vi "Import Export - Import from XML File.vi"(8 "error in":errorcluster, 10 "Configuration File Path":path, 11 "Item Ref in":T1 format="%.0x") -> (0 "error out":errorcluster, 3 "Item Ref out":T1 format="%.0x", 4 "xml string":string)   [LabVIEW 2017, in "Scan Engine Custom Device.lvlib"]
uses:
  Scan Engine Custom Device.lvlib
  <vilib>/NI Veristand/Custom Device API/Custom Device Item Ref.ctl
  <vilib>/NI/NI VeriStand Custom Device Import and Export Tool/ImportExport.lvlib
  <vilib>/NI Veristand/Custom Device API/Custom Device API.lvlib
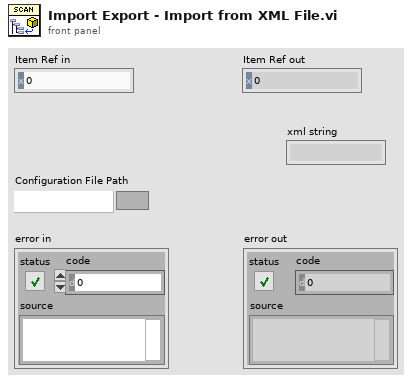
[diagram p1: front panel]
types:
  T1 = typedef "Custom Device API.lvlib/Custom Device Item Ref.ctl" = u64
  T2 = typedef "Advanced System Definition.lvlib/SysDef.Export.ctl" = cluster{"Version":string, "Tree":T3[]}
  T3 = typedef "Advanced System Definition.lvlib/TreeItem.ctl" = cluster{"Item Info":T4, "Parent Path":string[], "Properties":T9[]}
  T4 = typedef "Advanced System Definition.lvlib/TreeItem.Info.ctl" = cluster{"Name":string, "Description":string, "GUID":string, "Is Channel":bool, "Channel":T5, "Is Waveform":bool, "Waveform":T7}
  T5 = typedef "Custom Device API.lvlib/Custom Device Channel.ctl" = cluster{"Type":T6, "Units":string, "Default Value":dbl, "Faultable":bool, "Scalable":bool}
  T6 = typedef "Custom Device API.lvlib/Custom Device Channel Type.ctl" = enum16{"Input", "Output"}
  T7 = typedef "Custom Device API.lvlib/Custom Device Waveform.ctl" = cluster{"Data Type":T8, "Units":string}
  T8 = typedef "Custom Device API.lvlib/Custom Device Waveform DataType.ctl" = enum16{"Double", "Complex Double"}
  T9 = typedef "Advanced System Definition.lvlib/TreeItem.Property.ctl" = cluster{"Name":string, "Type":i32, "Value":variant}
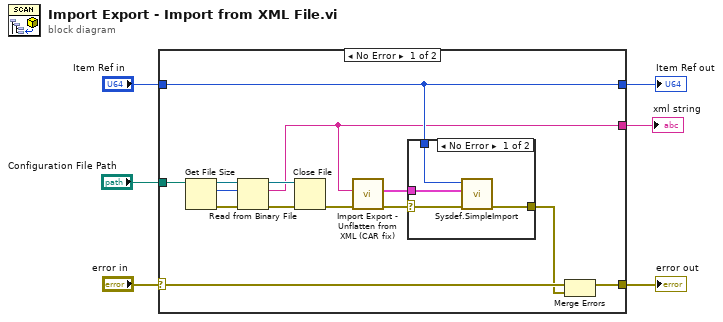
[diagram p0: block diagram]
diagram:
  n1 = case shown="No Error" "error in" {
    selector: "error in" -> [w20 w26]
    tunnel: [w17 w26] -> w5
    tunnel: [w19 w27] -> w4
    tunnel: "Item Ref in" -> [w19 w27]
    tunnel: "Configuration File Path" -> [w18 _]
    tunnel: [w10 _] -> w1
    frame No Error {
      n2 = Get File Size(file=w18) -> (refnum out=w14:refnum<file>, size (in bytes)=w15:i64, 0:w12:errorcluster)  [unwired: 1 in]
      n3 = Read from Binary File(8:w12, 10:w15, 11:w14) -> (0:w11:errorcluster, 2:w10:string, 3:w13:refnum<file>)  [unwired: 3 in, 1 out]
      n4 = Close File(refnum=w13, error in=w11) -> (error out=w8:errorcluster)  [unwired: 1 out]
      n5 = call "Import Export - Unflatten from XML (CAR fix).vi"("Error In"=w8, "XML String In"=w10) -> ("Error Out"=w9:errorcluster, "Import"=w7:T2)  [unwired: 8 in]
      n6 = case shown="No Error" w9 {
        selector: w9 -> [w23 w25]
        tunnel: w7 -> [w24 _]
        tunnel: [w22 w25] -> w16
        tunnel: w19 -> [w21 _]
        frame No Error {
          n7 = call <vilib>:"Sysdef.SimpleImport.vi"("error in (no error)"=w23, "SysDef"=w24, "NodeID"=w21) -> ("error out"=w22:errorcluster)  [unwired: 7 in, 1 out]
        }
        frame Error {
        }
      }
      n8 = Merge Errors(w20, w16) -> (w17:errorcluster)
    }
    frame Error {
    }
  }
  "error out" <- w5
  "Item Ref out" <- w4
  "xml string" <- w1
